vi "Initialize or Close Custom Instrument Sessions.vi"(0 "TSM Context":T1, 5 "Operation":enum16{"Initialize", "Close"}(ring), 11 "error in":errorcluster) -> (15 "error out":errorcluster)   [LabVIEW 2023, in "RFCalAndFixtureCharact.Common.lvlib"]
uses:
  RFCalAndFixtureCharact.Common.lvlib
  <vilib>/NI_TestStand_SemiconductorModule/NI_TestStand_Semiconductor_Module.lvlibp/PinMap/General/SemiconductorModuleContext.ctl
  <vilib>/NI_TestStand_SemiconductorModule/NI_TestStand_Semiconductor_Module.lvlibp
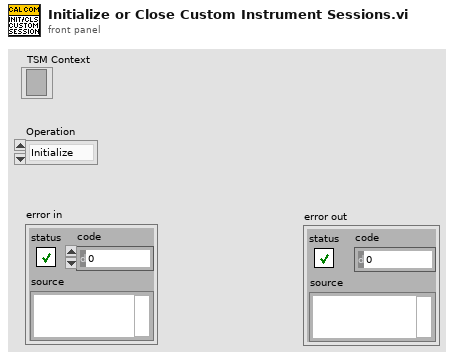
[diagram p1: front panel]
types:
  T1 = typedef "NI_TestStand_Semiconductor_Module.lvlibp/SemiconductorModuleContext.ctl" = refnum<k7>
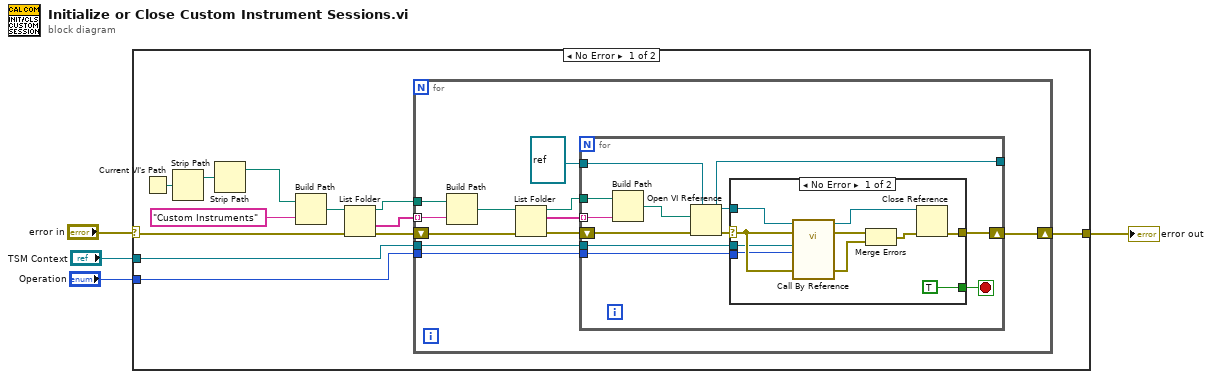
[diagram p0: block diagram]
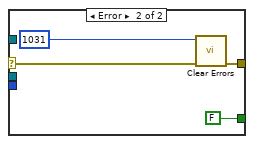
[diagram p2: hidden frame]
diagram:
  n1 = case shown="No Error" "error in" {
    selector: "error in" -> [w8 w53]
    tunnel: "TSM Context" -> [w7 _]
    tunnel: [w6 w53] -> w2
    tunnel: "Operation" -> [w5 _]
    frame No Error {
      n2 = Current VI's Path() -> (path=w15:path)
      n3 = Strip Path(path=w15) -> (stripped path=w16:path)  [unwired: 1 out]
      n4 = Strip Path(path=w16) -> (stripped path=w13:path)  [unwired: 1 out]
      n5 = Build Path(base path=w13, name or relative path="Custom Instruments") -> (appended path=w12:path)
      n6 = List Folder(path=w12, error in=w8) -> (path out=w9:path, folder names=w10:string[], error out=w11:errorcluster)  [unwired: 2 in, 1 out]
      n7 = for {
        shift-right: [w17] -> w6
        shift-left: w11 -> [w24]
        tunnel: w10 -> [w27] mode=indexing
        tunnel: w9 -> [w26]
        tunnel: w7 -> [w19]
        tunnel: w5 -> [w18]
        n8 = Build Path(base path=w26, name or relative path=w27) -> (appended path=w22:path)
        n9 = List Folder(path=w22, error in=w24) -> (path out=w20:path, filenames=w21:string[], error out=w23:errorcluster)  [unwired: 2 in, 1 out]
        n10 = for {
          tunnel: refnum<vi> refnum ("type specifier VI Refnum (for type only)") -> [w38]
          shift-right: [w32] -> w17
          shift-left: w23 -> [w37]
          tunnel: w21 -> [w36] mode=indexing
          tunnel: w20 -> [w35]
          tunnel: [w30] -> _
          tunnel: w19 -> [w29]
          tunnel: w18 -> [w28]
          stop <- w31 stop-if-true
          n11 = Build Path(base path=w35, name or relative path=w36) -> (appended path=w34:path)
          n12 = Open VI Reference(type specifier VI Refnum (for type only)=w38, vi path=w34, error in (no error)=w37) -> (vi reference=w30:refnum<vi>, error out=w33:errorcluster)  [unwired: 3 in]
          n13 = case shown="No Error" w33 {
            selector: w33 -> [w45 w51]
            tunnel: [w39 w52] -> w32
            tunnel: [TRUE FALSE] -> w31
            tunnel: w30 -> [w46 _]
            tunnel: w29 -> [w44 _]
            tunnel: w28 -> [w43 _]
            frame No Error {
              n14 = call-by-ref "?"(reference=w46, error in=w45, "TSM Context"=w44, "Operation"=w43, "error in"=w45) -> (reference out=w47:refnum<vi>, error out=w41:errorcluster, 15:"error out"=w42:errorcluster)  [unwired: 12 in]
              n15 = Merge Errors(w41, w42) -> (w40:errorcluster)
              n16 = Close Reference(reference=w47, error in (no error)=w40) -> (error out=w39:errorcluster)
            }
            frame Error {
              n17 = call <vilib>:"Clear Errors.vi"("error in (no error)"=w51, "specific error code to clear (0: all)"=1031 ("error code (0)")) -> ("error out"=w52:errorcluster)  [unwired: 4 in, 1 out]
            }
          }
        }
      }
    }
    frame Error {
    }
  }
  "error out" <- w2
